vi "update GUI.vi"(8 "error in (no error)":errorcluster, 11 "Autofocus in":refnum<class "Autofocus.lvclass">) -> (0 "error out":errorcluster, 3 "Autofocus out":refnum<class "Autofocus.lvclass">)   [LabVIEW 2012, in "Autofocus.lvclass"]
uses:
  Autofocus.lvclass
  Autofocus.lvclass/Autofocus.ctl
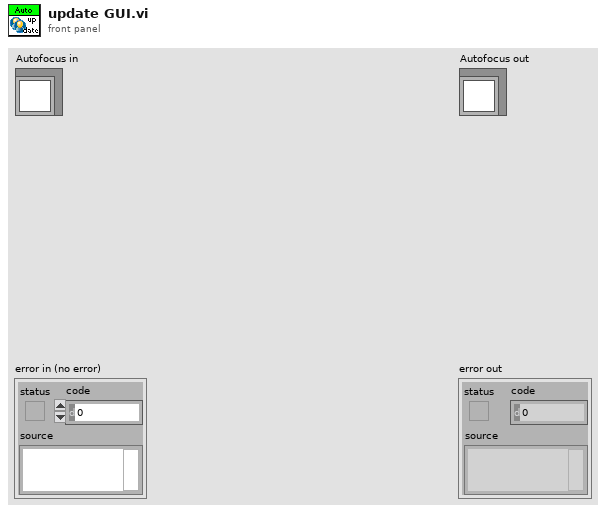
[diagram p1: front panel]
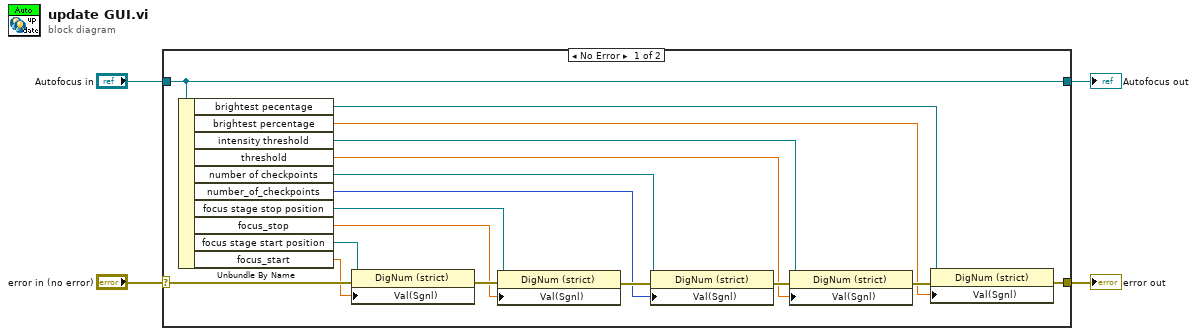
[diagram p0: block diagram]
diagram:
  n1 = case shown="No Error" "error in (no error)" {
    selector: "error in (no error)" -> [w20 w23]
    tunnel: [w5 w23] -> w3
    tunnel: [w21 w22] -> w1
    tunnel: "Autofocus in" -> [w21 w22]
    frame No Error {
      n2 = Unbundle By Name(w21) -> ("brightest pecentage"=w6:refnum<vi>, "brightest percentage"=w7:dbl, "intensity threshold"=w8:refnum<vi>, "threshold"=w9:dbl, "number of checkpoints"=w13:refnum<vi>, "number_of_checkpoints"=w12:u16, "focus stage stop position"=w16:refnum<vi>, "focus_stop"=w15:dbl[unit], "focus stage start position"=w18:refnum<vi>, "focus_start"=w19:dbl[unit])
      n3 = property class="DigNum (strict)"(reference=w18, error in=w20, "Val(Sgnl)"=w19) -> (error out=w17:errorcluster)  [unwired: 1 out]
      n4 = property class="DigNum (strict)"(reference=w16, error in=w17, "Val(Sgnl)"=w15) -> (error out=w14:errorcluster)  [unwired: 1 out]
      n5 = property class="DigNum (strict)"(reference=w13, error in=w14, "Val(Sgnl)"=w12) -> (error out=w11:errorcluster)  [unwired: 1 out]
      n6 = property class="DigNum (strict)"(reference=w8, error in=w11, "Val(Sgnl)"=w9) -> (error out=w10:errorcluster)  [unwired: 1 out]
      n7 = property class="DigNum (strict)"(reference=w6, error in=w10, "Val(Sgnl)"=w7) -> (error out=w5:errorcluster)  [unwired: 1 out]
    }
    frame Error {
    }
  }
  "error out" <- w3
  "Autofocus out" <- w1
